vi "Get Instr Identifier.vi"(8 "error in (no error)":errorcluster, 11 "Configuration Base in":refnum<class "CFG JSON Base.lvclass">) -> (0 "error out":errorcluster, 2 "Instr Identifier":string, 3 "Configuration Base out":refnum<class "CFG JSON Base.lvclass">)   [LabVIEW 2023, in "HAL GOOP4.lvlib" / "CFG JSON Base.lvclass"]
uses:
  CFG JSON Base.lvclass
  CFG JSON Base.lvclass/CFG JSON Base.ctl
  93c41ed1-0e68-4773-967c-815ca95f02ed.vi
  <vilib>/JDP Science/JSONtext/Find Item.vi
  <vilib>/JDP Science/JSONtext/Next JSON Value.vi
  <vilib>/JDP Science/JSONtext/String Subset.vi
  <vilib>/JDP Science/JSONtext/Parsing/Advance past next JSON Value (inlined COPY).vi
  <vilib>/JDP Science/JSONtext/Parsing/Advance past whitespace.vi
  <vilib>/JDP Science/JSONtext/Parsing/Advance past String.vi
  <vilib>/JDP Science/JSONtext/Parsing/Advance past Number.vi
  <vilib>/JDP Science/JSONtext/Parsing/Advance past Line Ending.vi
  <vilib>/JDP Science/JSONtext/Parsing/Parse Full Path or Item Name.vi
  <vilib>/JDP Science/JSONtext/Parsing/Advance past Array.vi
  <vilib>/JDP Science/JSONtext/Parsing/Advance past Object.vi
  <vilib>/JDP Science/JSONtext/support/Error Cluster From Code.vi
  <vilib>/JDP Science/JSONtext/Offset/Find Item Locations by Path.vi
  <vilib>/JDP Science/JSONtext/JSON text to Variant.vi
  <vilib>/Utility/error.llb/Error Cluster From Error Code.vi
  <vilib>/JDP Science/JSONtext/LVClass Serializer/JSONtext LVClass Serializer.lvclass
  <vilib>/ErrorRing/Error Ring.xnode
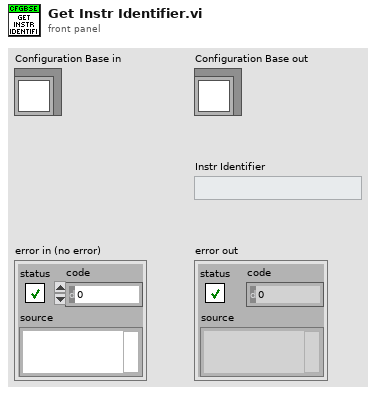
[diagram p1: front panel]
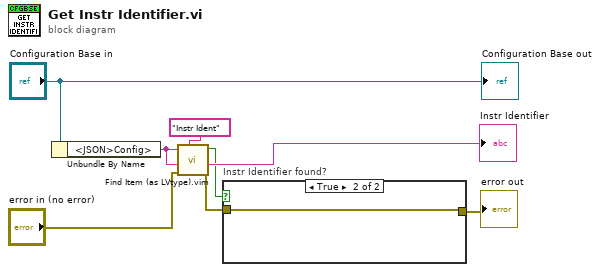
[diagram p0: block diagram]
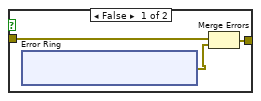
[diagram p2: hidden frame]
diagram:
  n1 = Unbundle By Name("Configuration Base in") -> ("<JSON>Config>"=w5:string)
  n2 = call "Find Item (as LVtype).vim"("$Path or Item Name"="Instr Ident", "error in (no error)"="error in (no error)", "Data Type and Default Value"=w5, "JSON"=w5) -> ("error out"=w2:errorcluster, "Data"=→"Instr Identifier":string, "Found"=w3:bool)  [unwired: 4 in, 1 out]
  n3 = case "Instr Identifier found?" shown="True" w3 {
    tunnel: w2 -> [w10 w17]
    tunnel: [w9 w17] -> w1
    frame False {
      n4 = xnode "Error Ring"() -> ("error out"=w11:errorcluster)
      n5 = Merge Errors(w10, w11) -> (w9:errorcluster)
    }
    frame True {
    }
  }
  "error out" <- w1
  "Configuration Base out" <- "Configuration Base in"
